vi "Add Paragraphs.vi"(8 "Error In":errorcluster, 11 "Multiple Newline Description":string) -> (0 "Error Out":errorcluster, 3 "Paragraph Description":string)   [LabVIEW 2018, in "Scripts.lvlib"]
uses:
  Scripts.lvlib
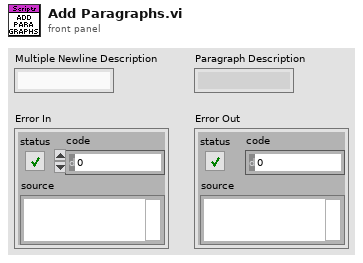
[diagram p1: front panel]
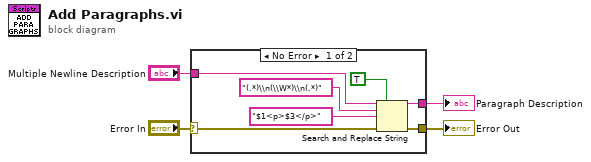
[diagram p0: block diagram]
diagram:
  n1 = case shown="No Error" "Error In" {
    selector: "Error In" -> [w5 w12]
    tunnel: [w11 _] -> w4
    tunnel: "Multiple Newline Description" -> [w10 _]
    tunnel: [w9 w12] -> w2
    frame No Error {
      n2 = Search and Replace String(replace all?=TRUE ("replace all? (F)"), input string=w10, search string="(.*)\\n(\\W*)\\n(.*)", replace string="$1<p>$3</p>" ("replace string (\"\")"), error in=w5) -> (result string=w11:string, error out=w9:errorcluster)  [unwired: 3 in, 2 out]
    }
    frame Error {
    }
  }
  "Paragraph Description" <- w4
  "Error Out" <- w2
